vi "VI References Storage.vi"(6 "Action":enum16{"Get", "Add/Replace", "Remove", "Clear"}(ring), 8 "Error In":errorcluster, 10 "VI Name":string, 11 "VI Refnum":refnum<vi>) -> (0 "Error Out":errorcluster, 1 "Front Panel Window:State":T1(ring), 3 "VI Refnum":refnum<vi>)   [LabVIEW 2021, in "GUI.lvlib"]
uses:
  GUI.lvlib
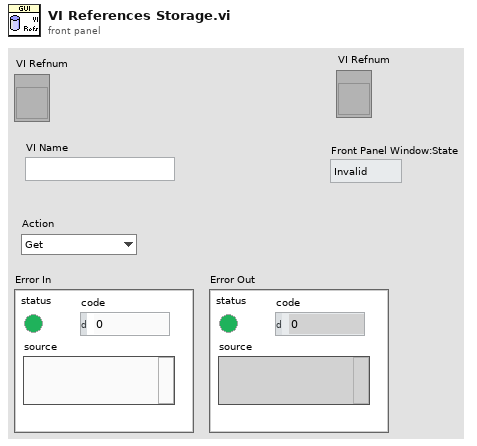
[diagram p1: front panel]
types:
  T1 = enum32{"Invalid", "Standard", "Closed", "Hidden", "Minimized", "Maximized"}
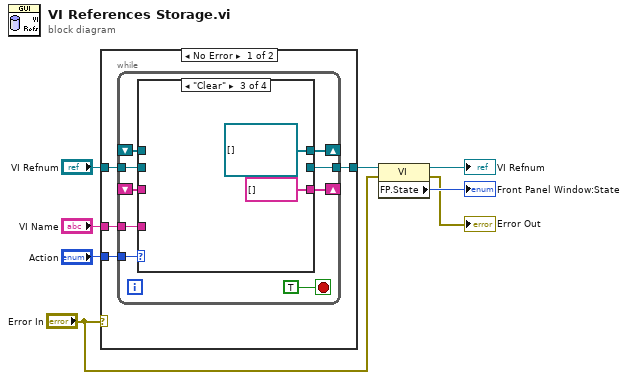
[diagram p0: block diagram]
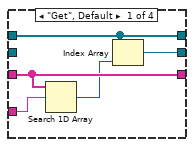
[diagram p2: hidden frame]
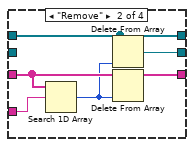
[diagram p3: hidden frame]
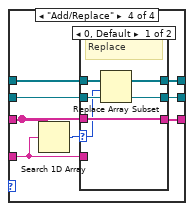
[diagram p4: hidden frame]
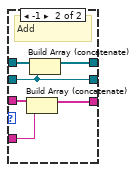
[diagram p5: hidden frame]
diagram:
  n1 = case shown="No Error" "Error In" {
    tunnel: "Action" -> [w12 _]
    tunnel: "VI Refnum" -> [w11 w54]
    tunnel: "VI Name" -> [w10 _]
    tunnel: [w9 w54] -> w5
    frame No Error {
      n2 = while {
        tunnel: w12 -> [w20]
        shift-right: [w14] -> _
        shift-left: _ -> [w15]
        shift-right: [w16] -> _
        shift-left: _ -> [w17]
        tunnel: w11 -> [w19]
        tunnel: w10 -> [w18]
        tunnel: [w13] -> w9
        stop <- TRUE stop-if-true
        n3 = case shown="\"Clear\"" w20 {
          tunnel: w19 -> [_ _ _ w37]
          tunnel: w18 -> [w26 w32 _ w41]
          tunnel: w17 -> [w25 w29 _ w40]
          tunnel: [w25 w27 string[] [] w39] -> w16
          tunnel: w15 -> [w22 w30 _ w38]
          tunnel: [w22 w30 refnum<vi>[] [] w36] -> w14
          tunnel: [w23 w31 _ w35] -> w13
          frame "Get", Default {
            n4 = Search 1D Array(1D array=w25, element=w26) -> (index of element=w24:i32)  [unwired: 1 in]
            n5 = Index Array(array=w22, index=w24) -> (element=w23:refnum<vi>)
          }
          frame "Remove" {
            n6 = Search 1D Array(1D array=w29, element=w32) -> (index of element=w28:i32)  [unwired: 1 in]
            n7 = Delete From Array(array=w30, index=w28) -> (deleted portion=w31:refnum<vi>)  [unwired: 1 in, 1 out]
            n8 = Delete From Array(array=w29, index=w28) -> (array with subset deleted=w27:string[])  [unwired: 1 in, 1 out]
          }
          frame "Clear" {
          }
          frame "Add/Replace" {
            n9 = Search 1D Array(1D array=w40, element=w41) -> (index of element=w42:i32)  [unwired: 1 in]
            n10 = case shown="0, Default" w42 {
              selector: w42 -> [w43 _]
              tunnel: w41 -> [_ w52]
              tunnel: w40 -> [w47 w53]
              tunnel: [w47 w51] -> w39
              tunnel: w38 -> [w46 w50]
              tunnel: w37 -> [w44 w48]
              tunnel: [w45 w49] -> w36
              tunnel: [w44 w48] -> w35
              frame 0, Default {
                # "Replace"
                n11 = Replace Array Subset(array=w46, new element=w44, index=w43) -> (w45:refnum<vi>[])
              }
              frame -1 {
                # "Add"
                n12 = Build Array (concatenate)(w53, w52) -> (w51:string[])
                n13 = Build Array (concatenate)(w50, w48) -> (w49:refnum<vi>[])
              }
            }
          }
        }
      }
    }
    frame Error {
    }
  }
  n14 = property class="VI"(reference=w5, error in="Error In") -> (reference out=→"VI Refnum":refnum<vi>, error out=→"Error Out":errorcluster, "FP.State"=→"Front Panel Window:State":T1)
